vi "Insertion Status.vi"() -> ()   [LabVIEW 2021]
uses:
  Controls/Insertion.ctl
panel:
  out "Insertion Status":T1
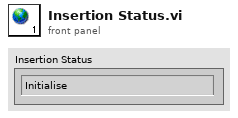
[diagram p1: front panel]
types:
  T1 = typedef "Insertion.ctl" = enum16{"Initialise", "Clamp Fwd", "Clamp Delay", "CYL Fwd", "Wait for Delay", "CYL Rear", "Done", "Error"}
diagram:
